vi "validate inputs.vi"(9 "output in":T3, 10 "process in":T1, 11 "input in":T2) -> (1 "output out":T3, 2 "process out":T1, 3 "input out":T2)   [LabVIEW 2013, in "data interface script.lvlib"]
uses:
  data interface script.lvlib
  Controls/output script control.ctl
  Controls/input script control.ctl
  Controls/processing script control.ctl
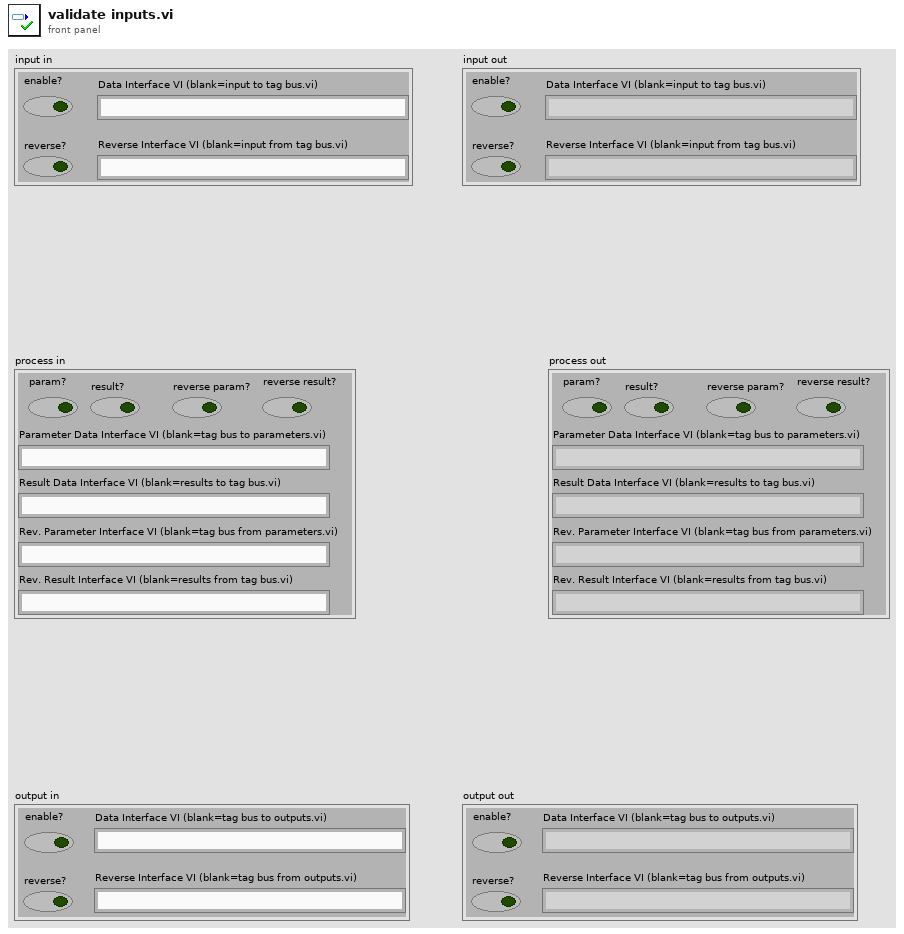
[diagram p1: front panel]
types:
  T1 = typedef "data interface script.lvlib/processing script control.ctl" = cluster{"param?":bool, "Parameter Data Interface VI (blank=tag bus to parameters.vi)":string, "Result Data Interface VI (blank=results to tag bus.vi)":string, "reverse param?":bool, "Rev. Result Interface VI (blank=results from tag bus.vi)":string, "Rev. Parameter Interface VI (blank=tag bus from parameters.vi)":string, "result?":bool, "reverse result?":bool}
  T2 = typedef "data interface script.lvlib/input script control.ctl" = cluster{"enable?":bool, "Data Interface VI (blank=input to tag bus.vi)":string, "reverse?":bool, "Reverse Interface VI (blank=input from tag bus.vi)":string}
  T3 = typedef "data interface script.lvlib/output script control.ctl" = cluster{"enable?":bool, "Data Interface VI (blank=tag bus to outputs.vi)":string, "Reverse Interface VI (blank=tag bus from outputs.vi)":string, "reverse?":bool}
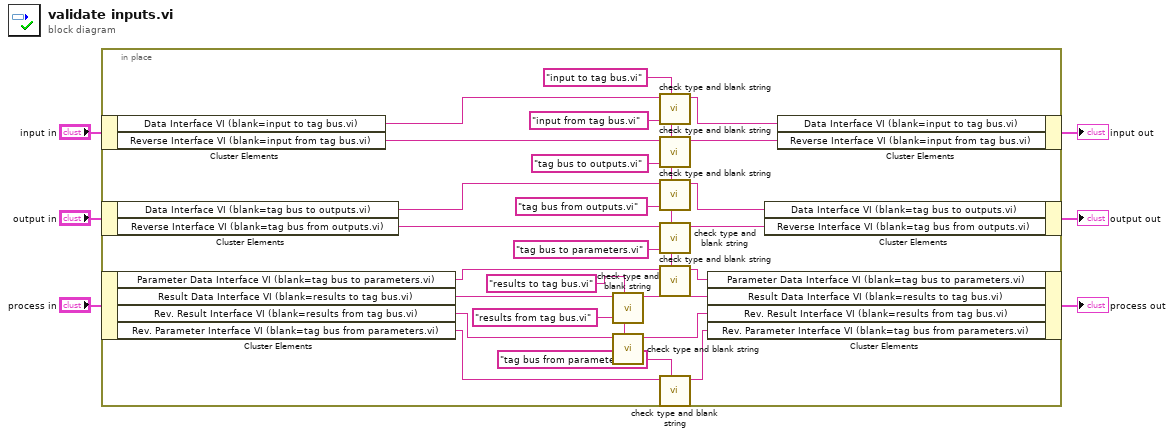
[diagram p0: block diagram]
diagram:
  n1 = in-place {
    n2 = in-place-cluster #1("input in") -> ("Data Interface VI (blank=input to tag bus.vi)"=w29:string, "Reverse Interface VI (blank=input from tag bus.vi)"=w16:string)
    n3 = in-place-cluster #2("output in") -> ("Data Interface VI (blank=tag bus to outputs.vi)"=w27:string, "Reverse Interface VI (blank=tag bus from outputs.vi)"=w8:string)
    n4 = in-place-cluster #3("process in") -> ("Parameter Data Interface VI (blank=tag bus to parameters.vi)"=w24:string, "Result Data Interface VI (blank=results to tag bus.vi)"=w23:string, "Rev. Result Interface VI (blank=results from tag bus.vi)"=w13:string, "Rev. Parameter Interface VI (blank=tag bus from parameters.vi)"=w10:string)
    n5 = call "check type and blank string.vi"("default"="results to tag bus.vi", "user input"=w23) -> ("validated"=w26:string)  [unwired: 9 in]
    n6 = call "check type and blank string.vi"("default"="results from tag bus.vi", "user input"=w13) -> ("validated"=w12:string)  [unwired: 9 in]
    n7 = call "check type and blank string.vi"("default"="input to tag bus.vi", "user input"=w29) -> ("validated"=w30:string)  [unwired: 9 in]
    n8 = call "check type and blank string.vi"("default"="input from tag bus.vi", "user input"=w16) -> ("validated"=w17:string)  [unwired: 9 in]
    n9 = call "check type and blank string.vi"("default"="tag bus to outputs.vi", "user input"=w27) -> ("validated"=w28:string)  [unwired: 9 in]
    n10 = call "check type and blank string.vi"("default"="tag bus from outputs.vi", "user input"=w8) -> ("validated"=w7:string)  [unwired: 9 in]
    n11 = call "check type and blank string.vi"("default"="tag bus to parameters.vi", "user input"=w24) -> ("validated"=w25:string)  [unwired: 9 in]
    n12 = call "check type and blank string.vi"("default"="tag bus from parameters.vi", "user input"=w10) -> ("validated"=w11:string)  [unwired: 9 in]
    n13 = in-place-cluster #3("Parameter Data Interface VI (blank=tag bus to parameters.vi)"=w25, "Result Data Interface VI (blank=results to tag bus.vi)"=w26, "Rev. Result Interface VI (blank=results from tag bus.vi)"=w12, "Rev. Parameter Interface VI (blank=tag bus from parameters.vi)"=w11) -> (→"process out":T1)
    n14 = in-place-cluster #2("Data Interface VI (blank=tag bus to outputs.vi)"=w28, "Reverse Interface VI (blank=tag bus from outputs.vi)"=w7) -> (→"output out":T3)
    n15 = in-place-cluster #1("Data Interface VI (blank=input to tag bus.vi)"=w30, "Reverse Interface VI (blank=input from tag bus.vi)"=w17) -> (→"input out":T2)
  }
